vi "Set Column Name.vi"(8 "error in (no error)":errorcluster, 10 "Column Name":string, 11 "Basic Column Configuration in":refnum<class "Basic Column Configuration.lvclass">) -> (0 "error out":errorcluster, 3 "Basic Column Configuration out":refnum<class "Basic Column Configuration.lvclass">)   [LabVIEW 2020, in "Basic Columns.lvlib" / "Basic Column Configuration.lvclass"]
uses:
  Basic Column Configuration.lvclass
  Basic Column Configuration.lvclass/Basic Column Configuration.ctl
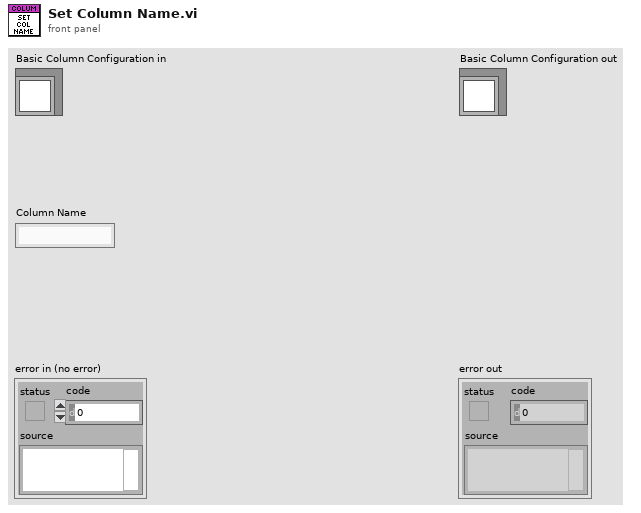
[diagram p1: front panel]
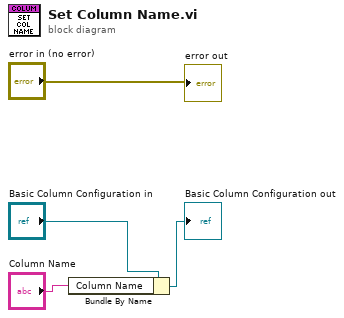
[diagram p0: block diagram]
diagram:
  n1 = Bundle By Name(cluster="Basic Column Configuration in", "Column Name"="Column Name") -> (→"Basic Column Configuration out":refnum<class "Basic Column Configuration.lvclass">)
  "error out" <- "error in (no error)"
